vi "dequeue.vi"(10 "memory ref":refnum<k21>, 11 "on-board buffer in":T1) -> (2 "data":u16, 3 "on-board buffer out":T1)   [LabVIEW 2010, in "OnBoardBuffer.lvlib"]
uses:
  OnBoardBuffer.lvlib
  buffer_state_cluster.ctl
  <vilib>/rvi/DataTransferAndStorage/Container/XNode/niFpgaContainer.xnode
  <vilib>/rvi/DataTransferAndStorage/Container/Common/niFpgaContainerMetaDataKey.ctl
  <vilib>/rvi/DataTransferAndStorage/Container/Common/niFpgaContainerExecOnDevCompGetState.vi
  <vilib>/rvi/Memory/Memory_Emulation/nirvimemoryEmulationManagerCache_GetValue.vi
  <vilib>/rvi/DataTransferAndStorage/Container/Common/niFpgaContainerGetUniqueNameForEmu.vi
  <vilib>/rvi/Memory/Memory_Emulation/nirvimemoryEmulationManagerCache_InsertValue.vi
  <vilib>/Utility/error.llb/Clear Errors.vi
  <vilib>/rvi/Memory/Memory_Emulation/nirvimemoryEmulationManagerCache_SetValue.vi
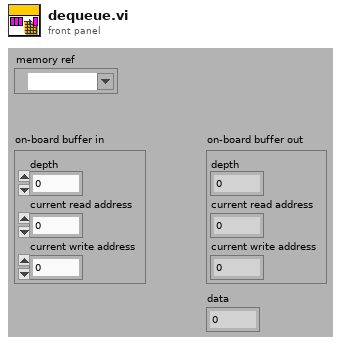
[diagram p1: front panel]
types:
  T1 = typedef "OnBoardBuffer.lvlib/buffer_state_cluster.ctl" = cluster{"depth":u32, "current read address":u32, "current write address":u32}
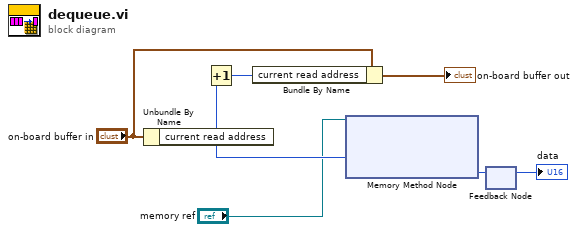
[diagram p0: block diagram]
diagram:
  n1 = Unbundle By Name("on-board buffer in") -> ("current read address"=w4:u32)
  n2 = Increment(x=w4) -> (x+1=w7:u32)
  n3 = Bundle By Name(cluster="on-board buffer in", "current read address"=w7) -> (→"on-board buffer out":T1)
  n4 = xnode ("Memory Method Node")("Address"=w4, "Memory In"="memory ref") -> ("Data"=w2:u16)  [unwired: 1 out]
  n5 = feedback-in #1(w2) -> ()
  n6 = feedback #1() -> (→"data":u16)  [unwired: 1 in]
